vi "Download Bitfile.vi"(8 "error in (no error)":errorcluster, 11 "starter kit FPGA host in":refnum<class "NI_Robotics_Starter Kit Host_FPGA_2.0.lvclass">) -> (0 "error out":errorcluster, 3 "starter kit FPGA host out":refnum<class "NI_Robotics_Starter Kit Host_FPGA_2.0.lvclass">)   [LabVIEW 2017, in "NI_Robotics_Starter Kit Host_FPGA_2.0.lvclass"]
uses:
  <vilib>/robotics/Starter Kit/2.0/FPGA Host Interface/NI_Robotics_Starter Kit Host_FPGA_2.0.lvclass
  <vilib>/robotics/Starter Kit/2.0/FPGA Host Interface/NI_Robotics_Starter Kit Host_FPGA_2.0.lvclass/NI_Robotics_Starter Kit Host_FPGA_2.0.ctl
  <vilib>/FPGAPlugInAG/Dynamic/niLvFpga_Download_Dynamic.vi
  <vilib>/robotics/Starter Kit/2.0/FPGA Host Interface/FPGA Refnum.ctl
  <vilib>/rvi/interface/nirviMethod/nirviMethod.xnode
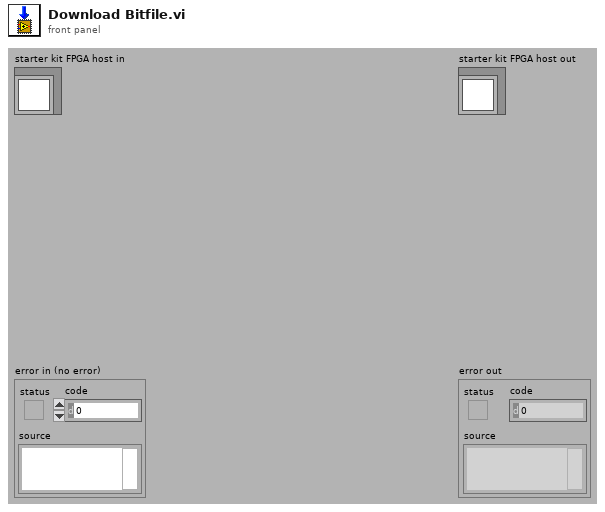
[diagram p1: front panel]
types:
  T1 = typedef "NI_Robotics_Starter Kit Host_FPGA_2.0.lvclass/FPGA Refnum.ctl" = refnum<k20>
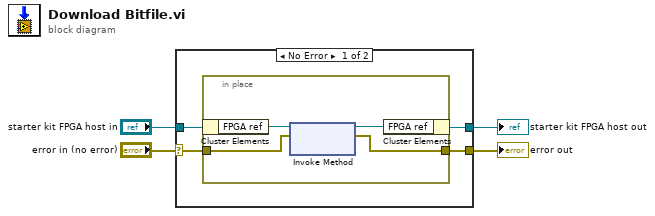
[diagram p0: block diagram]
diagram:
  n1 = case shown="No Error" "error in (no error)" {
    selector: "error in (no error)" -> [w5 w14]
    tunnel: "starter kit FPGA host in" -> [w8 w13]
    tunnel: [w7 w13] -> w1
    tunnel: [w6 w14] -> w2
    frame No Error {
      n2 = in-place {
        in-place-border: w5 -> [w10]
        in-place-border: [w9] -> w6
        n3 = in-place-cluster #1(w8) -> ("FPGA ref"=w12:T1)
        n4 = xnode "Invoke Method"("FPGA VI Reference In"=w12, "error in"=w10) -> ("FPGA VI Reference Out"=w11:T1, "error out"=w9:errorcluster)
        n5 = in-place-cluster #1("FPGA ref"=w11) -> (w7:refnum<class "NI_Robotics_Starter Kit Host_FPGA_2.0.lvclass">)
      }
    }
    frame Error {
    }
  }
  "error out" <- w2
  "starter kit FPGA host out" <- w1
